vi "Make Default Model.vi"(8 "error in (no error)":errorcluster) -> (0 "error out":errorcluster, 3 "Result Model out":refnum<class "Result Model.lvclass">)   [LabVIEW 2020, in "Result Model Statistics.lvclass"]
uses:
  Result Model Statistics.lvclass
  Framework/Result Model/Result Model.lvclass
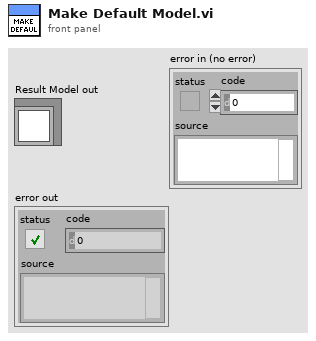
[diagram p1: front panel]
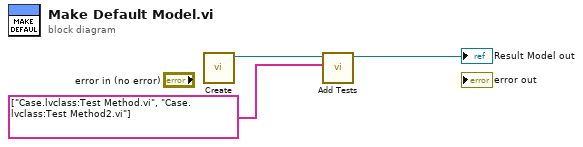
[diagram p0: block diagram]
diagram:
  n1 = call "Create.vi"() -> ("Result Model out"=w1:refnum<class "Result Model.lvclass">)  [unwired: 11 in]
  n2 = call "Add Tests.vi"("Tests"=string[] ["Case.lvclass:Test Method.vi", "Case.lvclass:Test Method2.vi"], "Result Model In"=w1) -> ("Result Model Out"=→"Result Model out":refnum<class "Result Model.lvclass">)  [unwired: 9 in]
